vi "Create Notifiers.vi"(8 "error in":errorcluster) -> (0 "error out":errorcluster, 3 "Notifiers":T1)   [LabVIEW 2014]
uses:
  Notifiers.ctl
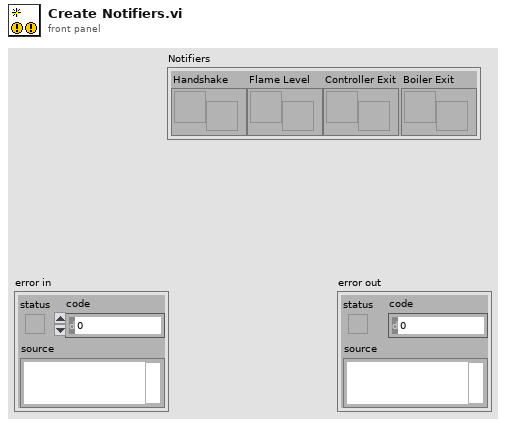
[diagram p1: front panel]
types:
  T1 = typedef "Notifiers.ctl" = cluster{"Handshake":refnum<notifier>, "Flame Level":refnum<notifier>, "Controller Exit":refnum<notifier>, "Boiler Exit":refnum<notifier>}
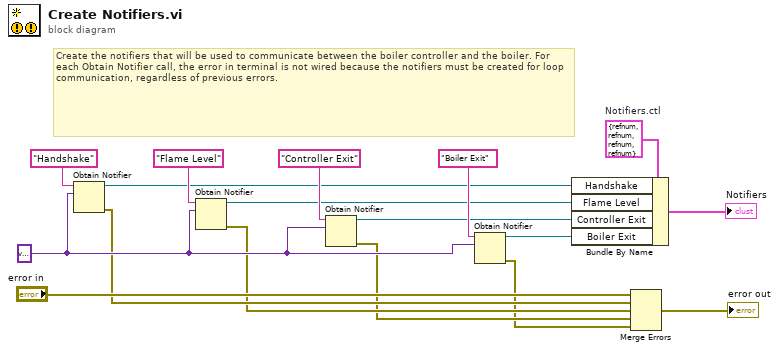
[diagram p0: block diagram]
diagram:
  w12 = T1 {"Handshake"=refnum, "Flame Level"=refnum, "Controller Exit"=refnum, "Boiler Exit"=refnum}  # Notifiers.ctl
  w14 = variant ("element data type")
  # "Create the notifiers that will be used to communicate between the boiler controller and the boiler. For each Obtain Notifier call, the error in terminal is not wired because the notifiers must be created for loop communication, regardless of previous errors."
  n1 = Obtain Notifier(name (unnamed)="Handshake", notification data type=w14) -> (notifier out=w8:refnum<notifier>, error out=w4:errorcluster)  [unwired: 2 in, 1 out]
  n2 = Obtain Notifier(name (unnamed)="Flame Level", notification data type=w14) -> (notifier out=w9:refnum<notifier>, error out=w3:errorcluster)  [unwired: 2 in, 1 out]
  n3 = Obtain Notifier(name (unnamed)="Controller Exit", notification data type=w14) -> (notifier out=w10:refnum<notifier>, error out=w2:errorcluster)  [unwired: 2 in, 1 out]
  n4 = Obtain Notifier(name (unnamed)="Boiler Exit", notification data type=w14) -> (notifier out=w11:refnum<notifier>, error out=w1:errorcluster)  [unwired: 2 in, 1 out]
  n5 = Bundle By Name(cluster=w12, "Handshake"=w8, "Flame Level"=w9, "Controller Exit"=w10, "Boiler Exit"=w11) -> (→"Notifiers":T1)
  n6 = Merge Errors("error in", w4, w3, w2, w1) -> (→"error out":errorcluster)
